vi "Teleop.vi"(10 "Match Info":T1={"Autonomous Elapsed Seconds"=0.0, "TeleOp Elapsed Seconds"=0.0, "Disabled Elapsed Seconds"=0.0, "Visited Autonomous"=FALSE, "Visited TeleOp"=FALSE, "Visited Disabled"=FALSE, "Autonomous Settings"={"Autonomous Style"=enum."Independent", "VI Refnum"=refnum}}, 11 "Call Context":T2) -> ()   [LabVIEW 2020]
doc: "This VI is called for each TeleOp packet received from the DS where the robot is not disabled. It is often used to read from the joysticks and update I/O or to update setpoints for timed control loops. It should complete and return within 20 milliseconds or it may miss DS packets."
uses:
  <vilib>/Rock Robotics/WPI/DriverStation/WPI_DriverStationDerivedRobotMode.ctl
  <vilib>/Rock Robotics/WPI/DriverStation/WPI_DriverStationMatch Info.ctl
  <vilib>/Rock Robotics/WPI/Joystick/XBox Axes Indexer.ctl
  <vilib>/Rock Robotics/WPI/ThirdParty/Phoenix-LabVIEW/Motor Controller/Controls/CTRE_Phoenix_MotorControl_ControlMode.ctl
  <vilib>/Rock Robotics/WPI/Utilities/WPI_GetSetVariantRefNum.vi
  <vilib>/Rock Robotics/Network Tables/NT Write Boolean Array.vi
  <vilib>/Rock Robotics/Network Tables/NT Write Numeric Array.vi
  <vilib>/Rock Robotics/Network Tables/NT Read Boolean.vi
  <vilib>/Rock Robotics/Network Tables/NT Read Number.vi
  <vilib>/Rock Robotics/WPI/ThirdParty/Phoenix-LabVIEW/Motor Controller/Get/CTRE_Phoenix_MotorController_GetSelectedSensorData.vi
panel:
  out "Voltage 4":dbl
  out "Voltage 3":dbl
  out "Voltage 2":dbl
  out "Voltage":dbl
  out "Sample Slider 0":dbl(slide) scale=0.0..5.0
  out "Sample Boolean 1":bool
  out "Sample Boolean 0":bool
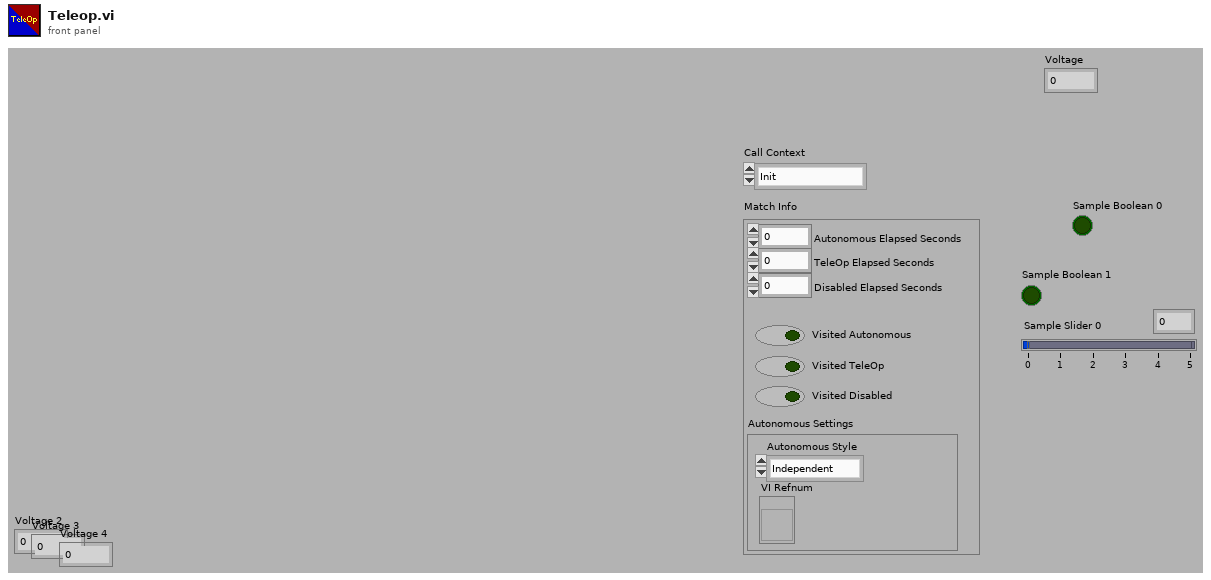
[diagram p1: front panel]
types:
  T1 = typedef "WPI_DriverStationMatch Info.ctl" = cluster{"Autonomous Elapsed Seconds":dbl, "TeleOp Elapsed Seconds":dbl, "Disabled Elapsed Seconds":dbl, "Visited Autonomous":bool, "Visited TeleOp":bool, "Visited Disabled":bool, "Autonomous Settings":cluster{"Autonomous Style":enum16{"Iterative", "Independent"}, "VI Refnum":refnum<vi>}}
  T2 = typedef "WPI_DriverStationDerivedRobotMode.ctl" = enum16{"Init", "Execute", "Stop"}
  T3 = typedef "CTRE_Phoenix_MotorControl_ControlMode.ctl" = u16
  T4 = typedef "XBox Axes Indexer.ctl" = enum16{"Left X", "Left Y", "Left Trigger", "Right Trigger", "Right X", "Right Y"}
  T5 = typedef "WPI_AnalogChannelDevRef.ctl" = cluster{"DevStatus":errorcluster, "Analog Channel":T6}
  T6 = typedef "FPGA_AIChannel.ctl" = enum8{"AI 0", "AI 1", "AI 2", "AI 3", "AI MXP 0", "AI MXP 1", "AI MXP 2", "AI MXP 3", "Invalid"}
  T7 = typedef "WPI_JoystickDevRef.ctl" = cluster{"Device":T8}
  T8 = typedef "WPI_JoystickDeviceEnum.ctl" = enum16{"USB 0", "USB 1", "USB 2", "USB 3", "USB 4", "USB 5"}
  T9 = typedef "WPI_MotorControlDeviceRef.ctl" = cluster{"DeviceStatus":errorcluster, "Type":T10, "PWM":cluster{"PWM Channel":T11, "DeadBand":T12}, "CAN":cluster{"Device Number":u8, "SetOutput VI Ref":variant, "GetOutput VI Ref":variant, "Enable VI Ref":variant, "Disable VI Ref":variant, "Data":variant}, "Invert":bool, "DIO PWM":cluster{"PWM \"Enable\" Channel":T11, "DIOChannel":T13, "PWM Rate":dbl}}
  T10 = typedef "WPI_MotorControlType.ctl" = enum16{"PWM", "CAN", "DIO PWM"}
  T11 = typedef "FPGA_DIOPWMChannel.ctl" = enum8{"PWM 0", "PWM 1", "PWM 2", "PWM 3", "PWM 4", "PWM 5", "PWM 6", "PWM 7", "PWM 8", "PWM 9", "PWM MXP 0", "PWM MXP 1", "PWM MXP 2", "PWM MXP 3", "PWM MXP 4", "PWM MXP 5", "PWM MXP 6", "PWM MXP 7", "PWM MXP 8", "PWM MXP 9", "Invalid"}
  T12 = typedef "WPI_PWMDeadband.ctl" = cluster{"Name":string, "maxPositivePwm":i32, "minPositivePwm":i32, "centerPwm":i32, "maxNegativePwm":i32, "minNegativePwm":i32, "angularRange":u16}
  T13 = typedef "FPGA_DIOChannel.ctl" = enum8{"DIO 0", "DIO 1", "DIO 2", "DIO 3", "DIO 4", "DIO 5", "DIO 6", "DIO 7", "DIO 8", "DIO 9", "DIO MXP 0", "DIO MXP 1", "DIO MXP 2", "DIO MXP 3", "DIO MXP 4", "DIO MXP 5", "DIO MXP 6", "DIO MXP 7", "DIO MXP 8", "DIO MXP 9", "DIO MXP 10", "DIO MXP 11", "DIO MXP 12", "DIO MXP 13", "DIO MXP 14", "DIO MXP 15", "SPI Port CS1", "SPI Port CS2", "SPI Port CS3", "SPI Port MISO", "SPI Port MOSI", "Invalid"}
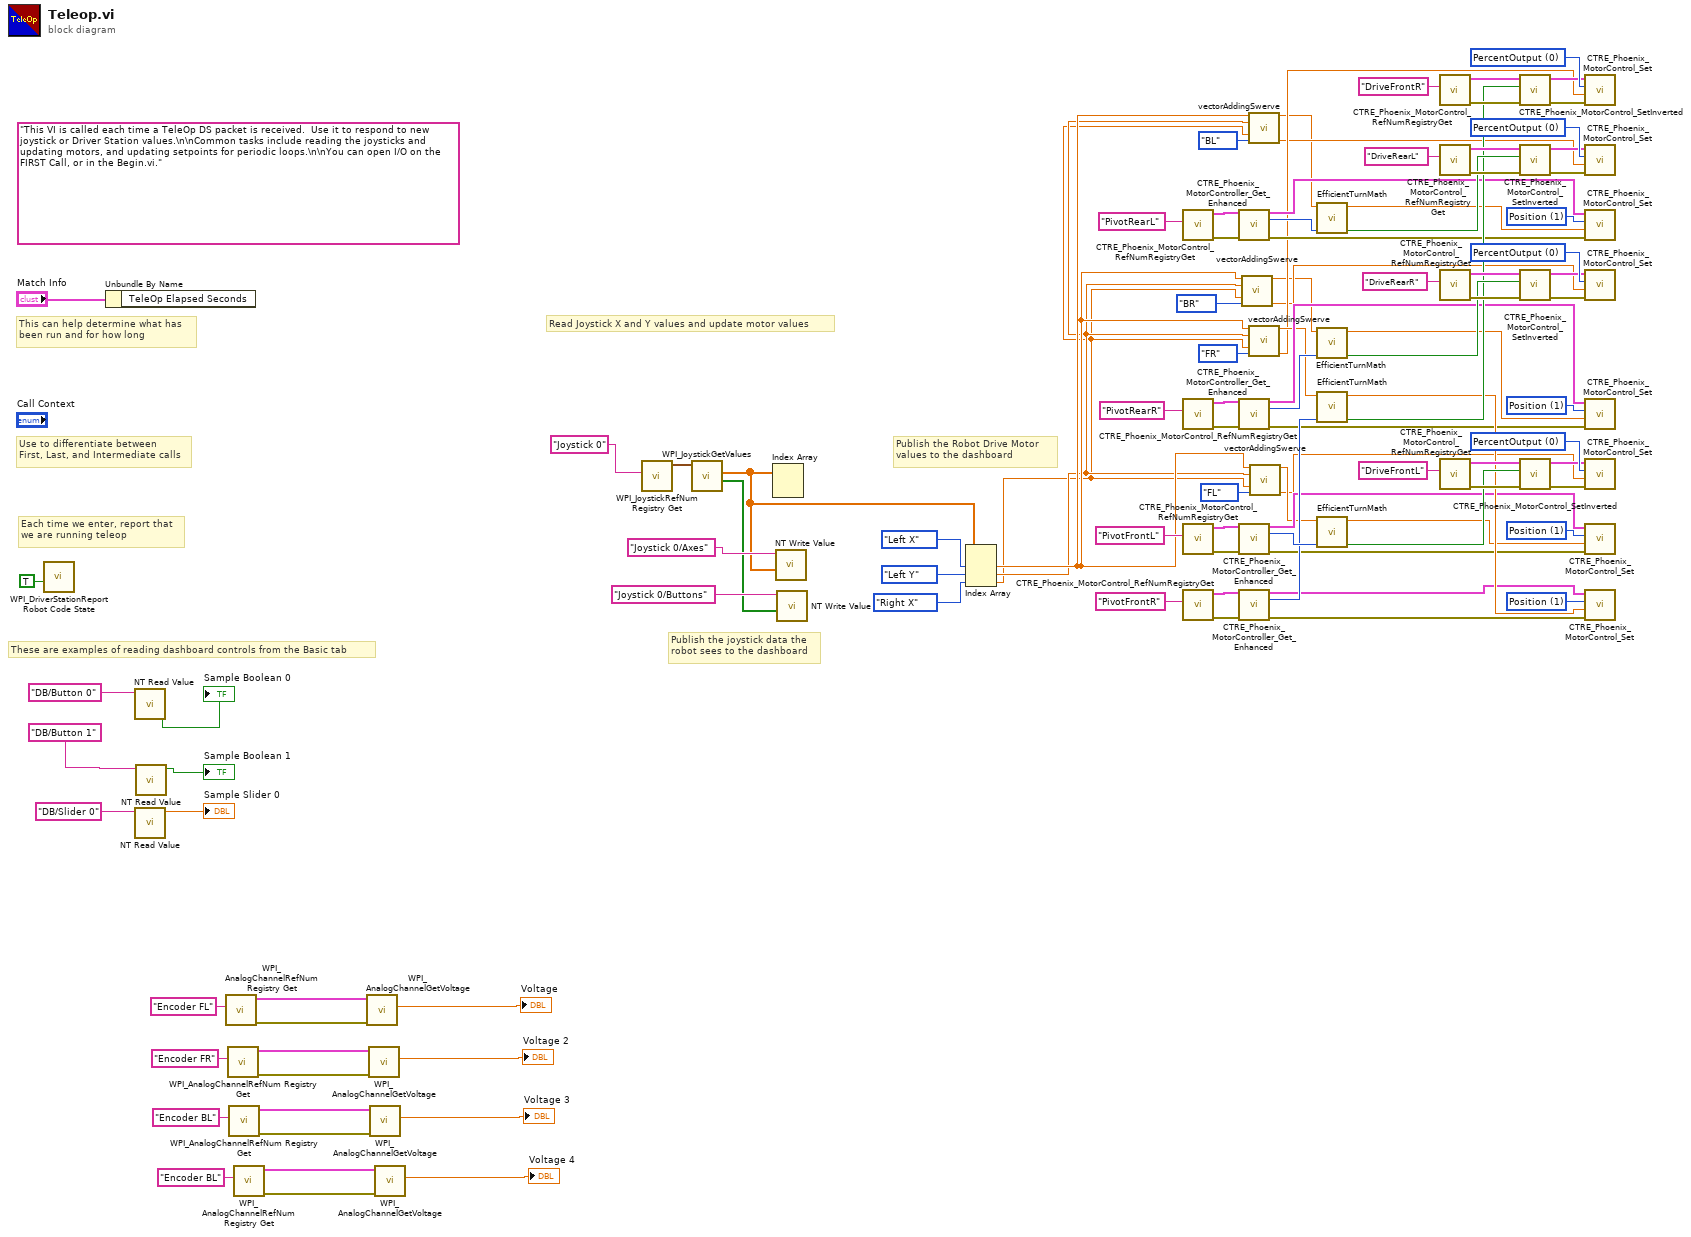
[diagram p0: block diagram]
diagram:
  w39 = T3 1 items=["PercentOutput"=0, "Position"=1, "Velocity"=2, "Current"=3, "Follower"=5, "MotionProfile"=6, "MotionMagic"=7, "MotionProfileArc"=10, "Disabled"=15] ("Control Mode")
  w40 = T3 1 items=["PercentOutput"=0, "Position"=1, "Velocity"=2, "Current"=3, "Follower"=5, "MotionProfile"=6, "MotionMagic"=7, "MotionProfileArc"=10, "Disabled"=15] ("Control Mode")
  w41 = T3 1 items=["PercentOutput"=0, "Position"=1, "Velocity"=2, "Current"=3, "Follower"=5, "MotionProfile"=6, "MotionMagic"=7, "MotionProfileArc"=10, "Disabled"=15] ("Control Mode")
  w43 = T3 1 items=["PercentOutput"=0, "Position"=1, "Velocity"=2, "Current"=3, "Follower"=5, "MotionProfile"=6, "MotionMagic"=7, "MotionProfileArc"=10, "Disabled"=15] ("Control Mode")
  w84 = T3 0 items=["PercentOutput"=0, "Position"=1, "Velocity"=2, "Current"=3, "Follower"=5, "MotionProfile"=6, "MotionMagic"=7, "MotionProfileArc"=10, "Disabled"=15] ("Control Mode")
  w85 = T3 0 items=["PercentOutput"=0, "Position"=1, "Velocity"=2, "Current"=3, "Follower"=5, "MotionProfile"=6, "MotionMagic"=7, "MotionProfileArc"=10, "Disabled"=15] ("Control Mode")
  w88 = T3 0 items=["PercentOutput"=0, "Position"=1, "Velocity"=2, "Current"=3, "Follower"=5, "MotionProfile"=6, "MotionMagic"=7, "MotionProfileArc"=10, "Disabled"=15] ("Control Mode")
  w89 = T3 0 items=["PercentOutput"=0, "Position"=1, "Velocity"=2, "Current"=3, "Follower"=5, "MotionProfile"=6, "MotionMagic"=7, "MotionProfileArc"=10, "Disabled"=15] ("Control Mode")
  (unwired) "This VI is called each time a TeleOp DS packet is received.  Use it to respond to new joystick or Driver Station values.\n\nCommon tasks include reading the joysticks and updating motors, and updating setpoints for periodic loops.\n\nYou can open I/O on the FIRST Call, or in the Begin.vi."
  # "These are examples of reading dashboard controls from the Basic tab"
  # "Publish the Robot Drive Motor\nvalues to the dashboard"
  # "Publish the joystick data the\nrobot sees to the dashboard"
  # "Each time we enter, report that\nwe are running teleop"
  # "Use to differentiate between\nFirst, Last, and Intermediate calls"
  # "This can help determine what has\nbeen run and for how long"
  # "Read Joystick X and Y values and update motor values"
  n1 = call <vilib>:"WPI_DriverStationReport Robot Code State.vi"("TeleOp"=TRUE ("Autonomous")) -> ()  [unwired: 10 in, 1 out]
  n2 = Unbundle By Name("Match Info") -> ()  [unwired: 1 out]
  n3 = call-poly <vilib>:"NT Read Value.vi"("Name"="DB/Button 0" ("refnum name")) -> ("Boolean"=→"Sample Boolean 0":bool)  [unwired: 9 in, 1 out]
  n4 = call-poly <vilib>:"NT Read Value.vi"("Name"="DB/Slider 0" ("refnum name")) -> ("Numeric"=→"Sample Slider 0":dbl)  [unwired: 9 in, 1 out]
  n5 = call-poly <vilib>:"NT Read Value.vi"("Name"="DB/Button 1" ("refnum name")) -> ("Boolean"=→"Sample Boolean 1":bool)  [unwired: 9 in, 1 out]
  n6 = call <vilib>:"WPI_AnalogChannelRefNum Registry Get.vi"("refnum name"="Encoder FL") -> ("error out"=w45:errorcluster, "AIDeviceRef"=w46:T5)  [unwired: 9 in]
  n7 = call <vilib>:"WPI_AnalogChannelRefNum Registry Get.vi"("refnum name"="Encoder FR") -> ("error out"=w10:errorcluster, "AIDeviceRef"=w11:T5)  [unwired: 9 in]
  n8 = call <vilib>:"WPI_AnalogChannelRefNum Registry Get.vi"("refnum name"="Encoder BL") -> ("error out"=w6:errorcluster, "AIDeviceRef"=w7:T5)  [unwired: 9 in]
  n9 = call <vilib>:"WPI_AnalogChannelRefNum Registry Get.vi"("refnum name"="Encoder BL") -> ("error out"=w2:errorcluster, "AIDeviceRef"=w3:T5)  [unwired: 9 in]
  n10 = call <vilib>:"WPI_AnalogChannelGetVoltage.vi"("error in (no error)"=w45, "AIDeviceRef"=w46) -> ("Voltage"=→"Voltage":dbl)  [unwired: 7 in, 2 out]
  n11 = call <vilib>:"WPI_AnalogChannelGetVoltage.vi"("error in (no error)"=w10, "AIDeviceRef"=w11) -> ("Voltage"=→"Voltage 2":dbl)  [unwired: 7 in, 2 out]
  n12 = call <vilib>:"WPI_AnalogChannelGetVoltage.vi"("error in (no error)"=w6, "AIDeviceRef"=w7) -> ("Voltage"=→"Voltage 3":dbl)  [unwired: 7 in, 2 out]
  n13 = call <vilib>:"WPI_AnalogChannelGetVoltage.vi"("error in (no error)"=w2, "AIDeviceRef"=w3) -> ("Voltage"=→"Voltage 4":dbl)  [unwired: 7 in, 2 out]
  n14 = call <vilib>:"WPI_JoystickRefNum Registry Get.vi"("refnum name"="Joystick 0") -> ("JoystickDevRef"=w106:T7)  [unwired: 1 in, 9 out]
  n15 = call <vilib>:"WPI_JoystickGetValues.vi"("JoystickDevRef"=w106) -> ("Buttons"=w102:bool[], "Axes"=w95:dbl[])  [unwired: 6 in, 3 out]
  n16 = Index Array(array=w95) -> ()  [unwired: 2 in, 2 out]
  n17 = call-poly <vilib>:"NT Write Value.vi"("Numeric Array"=w95, "Name"="Joystick 0/Axes") -> ()  [unwired: 9 in, 1 out]
  n18 = call-poly <vilib>:"NT Write Value.vi"("Boolean Array"=w102, "Name"="Joystick 0/Buttons") -> ()  [unwired: 9 in, 1 out]
  n19 = Index Array(array=w95, index #1=XBox_Axes_Indexer."Left X" ("XBox Axes"), index #2=XBox_Axes_Indexer."Left Y" ("XBox Axes"), index #3=XBox_Axes_Indexer."Right X" ("XBox Axes")) -> (element #1=w18:dbl, element #2=w17:dbl, element #3=w16:dbl)
  n20 = call <vilib>:"CTRE_Phoenix_MotorControl_RefNumRegistryGet.vi"("refnum name"="PivotRearL") -> ("error out"=w62:errorcluster, "PhoenixMotorControlDevRef"=w63:T9)  [unwired: 9 in]
  n21 = call <vilib>:"CTRE_Phoenix_MotorControl_RefNumRegistryGet.vi"("refnum name"="PivotRearR") -> ("error out"=w59:errorcluster, "PhoenixMotorControlDevRef"=w58:T9)  [unwired: 9 in]
  n22 = call <vilib>:"CTRE_Phoenix_MotorControl_RefNumRegistryGet.vi"("refnum name"="PivotFrontL") -> ("error out"=w65:errorcluster, "PhoenixMotorControlDevRef"=w66:T9)  [unwired: 9 in]
  n23 = call <vilib>:"CTRE_Phoenix_MotorControl_RefNumRegistryGet.vi"("refnum name"="PivotFrontR") -> ("error out"=w56:errorcluster, "PhoenixMotorControlDevRef"=w55:T9)  [unwired: 9 in]
  n24 = call-poly <vilib>:"CTRE_Phoenix_MotorController_Get_Enhanced.vi"("PhoenixMotorControlDevRef"=w63, "error in"=w62) -> ("PhoenixMotorControlDevRef"=w32:T9, "Position (Raw Sensor Units)"=w61:i32, "error out"=w28:errorcluster)  [unwired: 10 in, 1 out]
  n25 = call-poly <vilib>:"CTRE_Phoenix_MotorController_Get_Enhanced.vi"("PhoenixMotorControlDevRef"=w58, "error in"=w59) -> ("PhoenixMotorControlDevRef"=w33:T9, "Position (Raw Sensor Units)"=w60:i32, "error out"=w31:errorcluster)  [unwired: 10 in, 1 out]
  n26 = call-poly <vilib>:"CTRE_Phoenix_MotorController_Get_Enhanced.vi"("PhoenixMotorControlDevRef"=w66, "error in"=w65) -> ("PhoenixMotorControlDevRef"=w34:T9, "Position (Raw Sensor Units)"=w64:i32, "error out"=w30:errorcluster)  [unwired: 10 in, 1 out]
  n27 = call-poly <vilib>:"CTRE_Phoenix_MotorController_Get_Enhanced.vi"("PhoenixMotorControlDevRef"=w55, "error in"=w56) -> ("PhoenixMotorControlDevRef"=w35:T9, "Position (Raw Sensor Units)"=w57:i32, "error out"=w29:errorcluster)  [unwired: 10 in, 1 out]
  n28 = call "vectorAddingSwerve.vi"("LeftX"=w18, "LeftY"=w17, "RightX"=w16, "Wheel"=enum16{"FL", "FR", "BL", "BR"}."BR") -> ("Angle"=w19:dbl, "Magnitude"=w20:dbl)  [unwired: 10 in]
  n29 = call "vectorAddingSwerve.vi"("LeftX"=w18, "LeftY"=w17, "RightX"=w16, "Wheel"=enum16{"FL", "FR", "BL", "BR"}."BL") -> ("Angle"=w13:dbl, "Magnitude"=w14:dbl)  [unwired: 10 in]
  n30 = call "vectorAddingSwerve.vi"("LeftX"=w18, "LeftY"=w17, "RightX"=w16, "Wheel"=enum16{"FL", "FR", "BL", "BR"}."FR") -> ("Angle"=w25:dbl, "Magnitude"=w24:dbl)  [unwired: 10 in]
  n31 = call "vectorAddingSwerve.vi"("LeftX"=w18, "LeftY"=w17, "RightX"=w16, "Wheel"=enum16{"FL", "FR", "BL", "BR"}."FL") -> ("Angle"=w23:dbl, "Magnitude"=w22:dbl)  [unwired: 10 in]
  n32 = call "EfficientTurnMath.vi"("current"=w61, "target"=w13) -> ("Invert"=w49:bool, "AngleToTurn"=w42:dbl)  [unwired: 8 in]
  n33 = call "EfficientTurnMath.vi"("current"=w60, "target"=w19) -> ("Invert"=w48:bool, "AngleToTurn"=w36:dbl)  [unwired: 8 in]
  n34 = call "EfficientTurnMath.vi"("current"=w57, "target"=w25) -> ("Invert"=w47:bool, "AngleToTurn"=w38:dbl)  [unwired: 8 in]
  n35 = call "EfficientTurnMath.vi"("current"=w64, "target"=w23) -> ("Invert"=w50:bool, "AngleToTurn"=w37:dbl)  [unwired: 8 in]
  n36 = call <vilib>:"CTRE_Phoenix_MotorControl_RefNumRegistryGet.vi"("refnum name"="DriveFrontR") -> ("error out"=w68:errorcluster, "PhoenixMotorControlDevRef"=w70:T9)  [unwired: 9 in]
  n37 = call <vilib>:"CTRE_Phoenix_MotorControl_RefNumRegistryGet.vi"("refnum name"="DriveRearL") -> ("error out"=w81:errorcluster, "PhoenixMotorControlDevRef"=w82:T9)  [unwired: 9 in]
  n38 = call <vilib>:"CTRE_Phoenix_MotorControl_RefNumRegistryGet.vi"("refnum name"="DriveRearR") -> ("error out"=w76:errorcluster, "PhoenixMotorControlDevRef"=w78:T9)  [unwired: 9 in]
  n39 = call <vilib>:"CTRE_Phoenix_MotorControl_RefNumRegistryGet.vi"("refnum name"="DriveFrontL") -> ("error out"=w72:errorcluster, "PhoenixMotorControlDevRef"=w74:T9)  [unwired: 9 in]
  n40 = call <vilib>:"CTRE_Phoenix_MotorControl_SetInverted.vi"("error in (no error)"=w68, "Invert?"=w47, "PhoenixMotorControlDevRef"=w70) -> ("error out"=w67:errorcluster, "PhoenixMotorControlDevRef"=w69:T9)  [unwired: 7 in]
  n41 = call <vilib>:"CTRE_Phoenix_MotorControl_SetInverted.vi"("error in (no error)"=w81, "Invert?"=w49, "PhoenixMotorControlDevRef"=w82) -> ("error out"=w79:errorcluster, "PhoenixMotorControlDevRef"=w80:T9)  [unwired: 7 in]
  n42 = call <vilib>:"CTRE_Phoenix_MotorControl_SetInverted.vi"("error in (no error)"=w76, "Invert?"=w48, "PhoenixMotorControlDevRef"=w78) -> ("error out"=w75:errorcluster, "PhoenixMotorControlDevRef"=w77:T9)  [unwired: 7 in]
  n43 = call <vilib>:"CTRE_Phoenix_MotorControl_SetInverted.vi"("error in (no error)"=w72, "Invert?"=w50, "PhoenixMotorControlDevRef"=w74) -> ("error out"=w71:errorcluster, "PhoenixMotorControlDevRef"=w73:T9)  [unwired: 7 in]
  n44 = call <vilib>:"CTRE_Phoenix_MotorControl_Set.vi"("error in (no error)"=w67, "Output"=w24, "Control Mode"=w84, "PhoenixMotorControlDevRef"=w69) -> ()  [unwired: 6 in, 2 out]
  n45 = call <vilib>:"CTRE_Phoenix_MotorControl_Set.vi"("error in (no error)"=w79, "Output"=w14, "Control Mode"=w89, "PhoenixMotorControlDevRef"=w80) -> ()  [unwired: 6 in, 2 out]
  n46 = call <vilib>:"CTRE_Phoenix_MotorControl_Set.vi"("error in (no error)"=w28, "Output"=w42, "Control Mode"=w43, "PhoenixMotorControlDevRef"=w32) -> ()  [unwired: 6 in, 2 out]
  n47 = call <vilib>:"CTRE_Phoenix_MotorControl_Set.vi"("error in (no error)"=w75, "Output"=w20, "Control Mode"=w88, "PhoenixMotorControlDevRef"=w77) -> ()  [unwired: 6 in, 2 out]
  n48 = call <vilib>:"CTRE_Phoenix_MotorControl_Set.vi"("error in (no error)"=w31, "Output"=w36, "Control Mode"=w41, "PhoenixMotorControlDevRef"=w33) -> ()  [unwired: 6 in, 2 out]
  n49 = call <vilib>:"CTRE_Phoenix_MotorControl_Set.vi"("error in (no error)"=w71, "Output"=w22, "Control Mode"=w85, "PhoenixMotorControlDevRef"=w73) -> ()  [unwired: 6 in, 2 out]
  n50 = call <vilib>:"CTRE_Phoenix_MotorControl_Set.vi"("error in (no error)"=w30, "Output"=w37, "Control Mode"=w40, "PhoenixMotorControlDevRef"=w34) -> ()  [unwired: 6 in, 2 out]
  n51 = call <vilib>:"CTRE_Phoenix_MotorControl_Set.vi"("error in (no error)"=w29, "Output"=w38, "Control Mode"=w39, "PhoenixMotorControlDevRef"=w35) -> ()  [unwired: 6 in, 2 out]
